vi "Set_Speed_Command.vi"(1 "Speed Control":i16(slide) scale=0.0..4500.0) -> (0 "Speed Control String to send:":string)   [LabVIEW 2019]
doc: "This vi sends to inverter a new set speed value.\n**************************************\nDO NOT SEND A NEW SET SPEED VALUE UNLESS SERIAL COMMUNICATION IS CONTROLLING SET SPEED.\n**************************************"
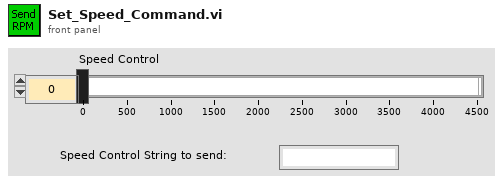
[diagram p1: front panel]
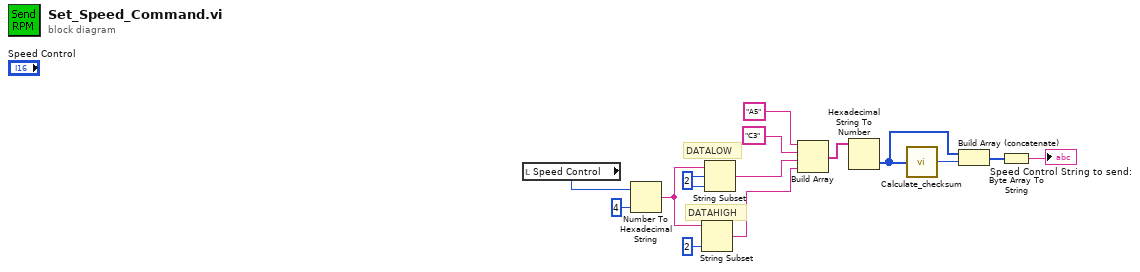
[diagram p0: block diagram]
diagram:
  w11 = 2 ("length (rest)")
  # "DATALOW"
  # "DATAHIGH"
  n1 = local read "Speed Control"() -> (w13:i16)
  n2 = Number To Hexadecimal String(1:i16 4 ("width (-)"), 2:w13) -> (0:w10:string)
  n3 = String Subset(string=w10, length (rest)=2 ("length (rest)")) -> (substring=w6:string)  [unwired: 1 in]
  n4 = String Subset(string=w10, offset (0)=w11, length (rest)=w11) -> (substring=w7:string)
  n5 = Build Array("A5", "C3", w7, w6) -> (w5:string[])
  n6 = Hexadecimal String To Number(string=w5) -> (number=w4:u32[])  [unwired: 2 in, 1 out]
  n7 = call "Calculate_checksum.vi"("Data"=w4) -> ("Checksum"=w3:i32)
  n8 = Build Array (concatenate)(w4, w3) -> (w2:u32[])
  n9 = Byte Array To String(unsigned byte array=w2) -> (string=→"Speed Control String to send:":string)
